vi "Check Closed.vi"() -> (0 "Closed?":bool)   [LabVIEW 2022 SP3, in "FlexBlocks Support.lvlib"]
uses:
  FlexBlocks Support.lvlib
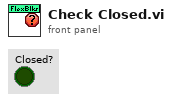
[diagram p1: front panel]
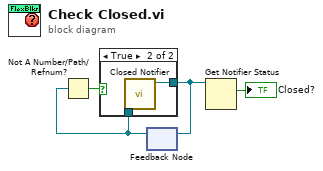
[diagram p0: block diagram]
diagram:
  n1 = feedback #1() -> (w3:refnum<notifier>)  [unwired: 1 in]
  n2 = Not A Number/Path/Refnum?(number/path/refnum=w3) -> (NaN/Path/Refnum?=w4:bool)
  n3 = case shown="True" w4 {
    tunnel: [w5 w6] -> w2
    tunnel: w3 -> [w5 _]
    frame False {
    }
    frame True {
      n4 = call "Closed Notifier.vi"() -> ("Closed Notifier"=w6:refnum<notifier>)  [unwired: 11 in]
    }
  }
  n5 = feedback-in #1(w2) -> ()
  n6 = Get Notifier Status(notifier=w2) -> (current notification=→"Closed?":bool)  [unwired: 1 in, 4 out]
